vi "TestTactic.vi"(8 "error in (no error)":errorcluster, 9 "Game in":refnum<class "Game.lvclass">, 10 "Robot":refnum<class "Robot.lvclass">, 11 "Tactic in":refnum<class "TestTactic.lvclass">) -> (0 "error out":errorcluster, 2 "Robot out":refnum<class "Robot.lvclass">, 3 "Tactic out":refnum<class "TestTactic.lvclass">)   [LabVIEW 2023, in "TestTactic.lvclass"]
uses:
  TestTactic.lvclass
  C:/Users/ebert/Documents/codes/SSL/repo/SSL_AI/Tactic_class/Tactic.lvclass
  Robot_class/Robot.lvclass
  Game_class/Game.lvclass
  Robot_class/tactics.ctl
  STP_Parameters/TestSkills.ctl
  Tactic_class/Tactic.lvclass/Tactic.ctl
  Game_class/Game.lvclass/Game.ctl
  Team_class/Team.lvclass/Team.ctl
  Robot_class/Robot.lvclass/Robot.ctl
  Game_class/Read BallRef.vi
  Game_class/Read EnemyRef.vi
  Team_class/Read RobotRef.vi
  Tactic_class/Read Skillbook.vi
  Robot_class/Write tactic.vi
  Enemy_class/Enemy.lvclass
  C:/Users/ebert/Documents/codes/SSL/repo/SSL_AI/Team_class/Team.lvclass
  Skillbook_class/Skillbook.lvclass
  Ball_class/Ball.lvclass
  Circulate_class/CirculateSkill.lvclass
  PassSkill_class/PassSkill.lvclass
  OneTouchShotSkill_class/OneTouchShotSkill.lvclass
  AlignSkill/AlignSkill.lvclass
  GoToSkill_v2_class/GoToSkill_v2.lvclass
panel:
  out "x .or. y?":bool
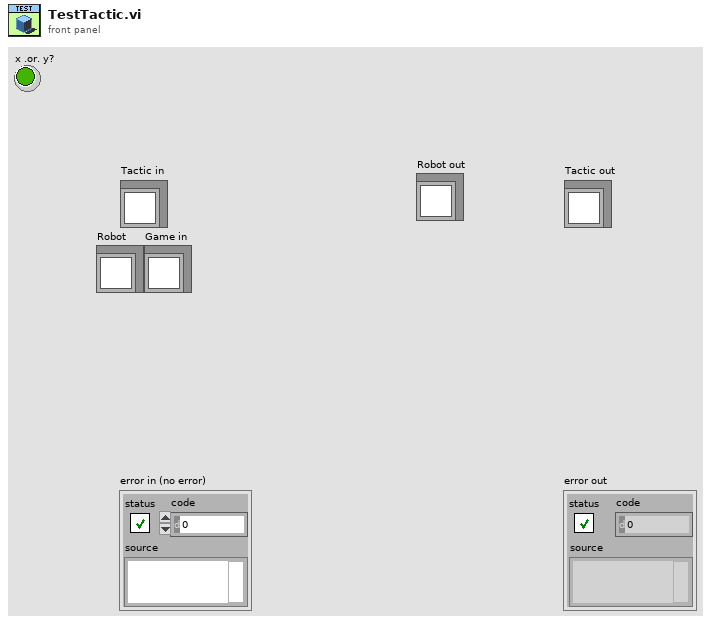
[diagram p1: front panel]
types:
  T1 = typedef "TestSkills.ctl" = enum16{"AlignSkill", "PassSkill", "CirculateBall", "OneTouchShotSkill", "KickToSkill_v2", "ShootSkill", "InterceptBall", "Exit", "GoToSkill_v2"}
  T2 = typedef "tactics.ctl" = enum16{"GoToBallPlacementPosition", "PlaceBall", "GoToBallPlacement", "5Robots", "BallPlacementEnemy", "ReceivePassInFuturePoint", "Roller", "PrepareRollToPassRollerGoTo", "PrepareRollToPassReceiverGoTo", "WaitRoll", "PositionToRoll", "PenaltyAttacker", "PassObserver", "PenaltyDefense", "TableReceiverTactic", "Test", "DefendGoal", "Marker", "FollowAttacker", "DefendArea", "Shoot", "AttackerAimGoal", "AttackerBallOutOfField", "AttackerBlock", "AttackerStop", "Duelist", "Halt", "ZigZag", "GoTo", "Timeout", "KickToBestRobot", "KickToPassReceiver", "PositionToReceivePass", "WaitPass"}
  T3 = typedef "STPParameters.ctl" = cluster{"Skills":T4, "TestSkill":T1, "Events":cluster{"distanceToBallPossession":dbl, "timeForPossessionThreshold":dbl}, "Criteria":cluster{"OpenAngleToGoal":cluster{"minAngle":dbl, "maxAngle":dbl, "minEvaluation":dbl}, "PassDistance":cluster{"maxDistance":dbl, "minDistance":dbl}, "ShotTime":cluster{"shotSpeed":dbl, "keeperSpeed":dbl, "maxShotDistance":dbl, "minEvaluation":dbl}, "OneTouchShot":cluster{"MaxAngle":dbl, "minEvaluation":dbl}, "BallInterception":cluster{"minEnemySpeed":dbl, "maxEnemySpeed":dbl, "chipPassDistance":dbl, "chipPassEval":dbl, "minEvaluation":dbl}}, "minPassSpeed":dbl, "maxPassSpeed":dbl, "AllyTeamIds":T6[]}
  T4 = typedef "Skills.ctl" = cluster{"CirculateBall":T5, "ProtectBall":cluster{"DistanceFromBall":dbl}}
  T5 = typedef "CIrculateSkillParameters.ctl" = cluster{"rotationAngle":dbl, "velocityFactor":dbl, "OrientationFactor":dbl}
  T6 = typedef "AllyTeam.ctl" = enum16{"Keeper", "Defender", "Attacker"}
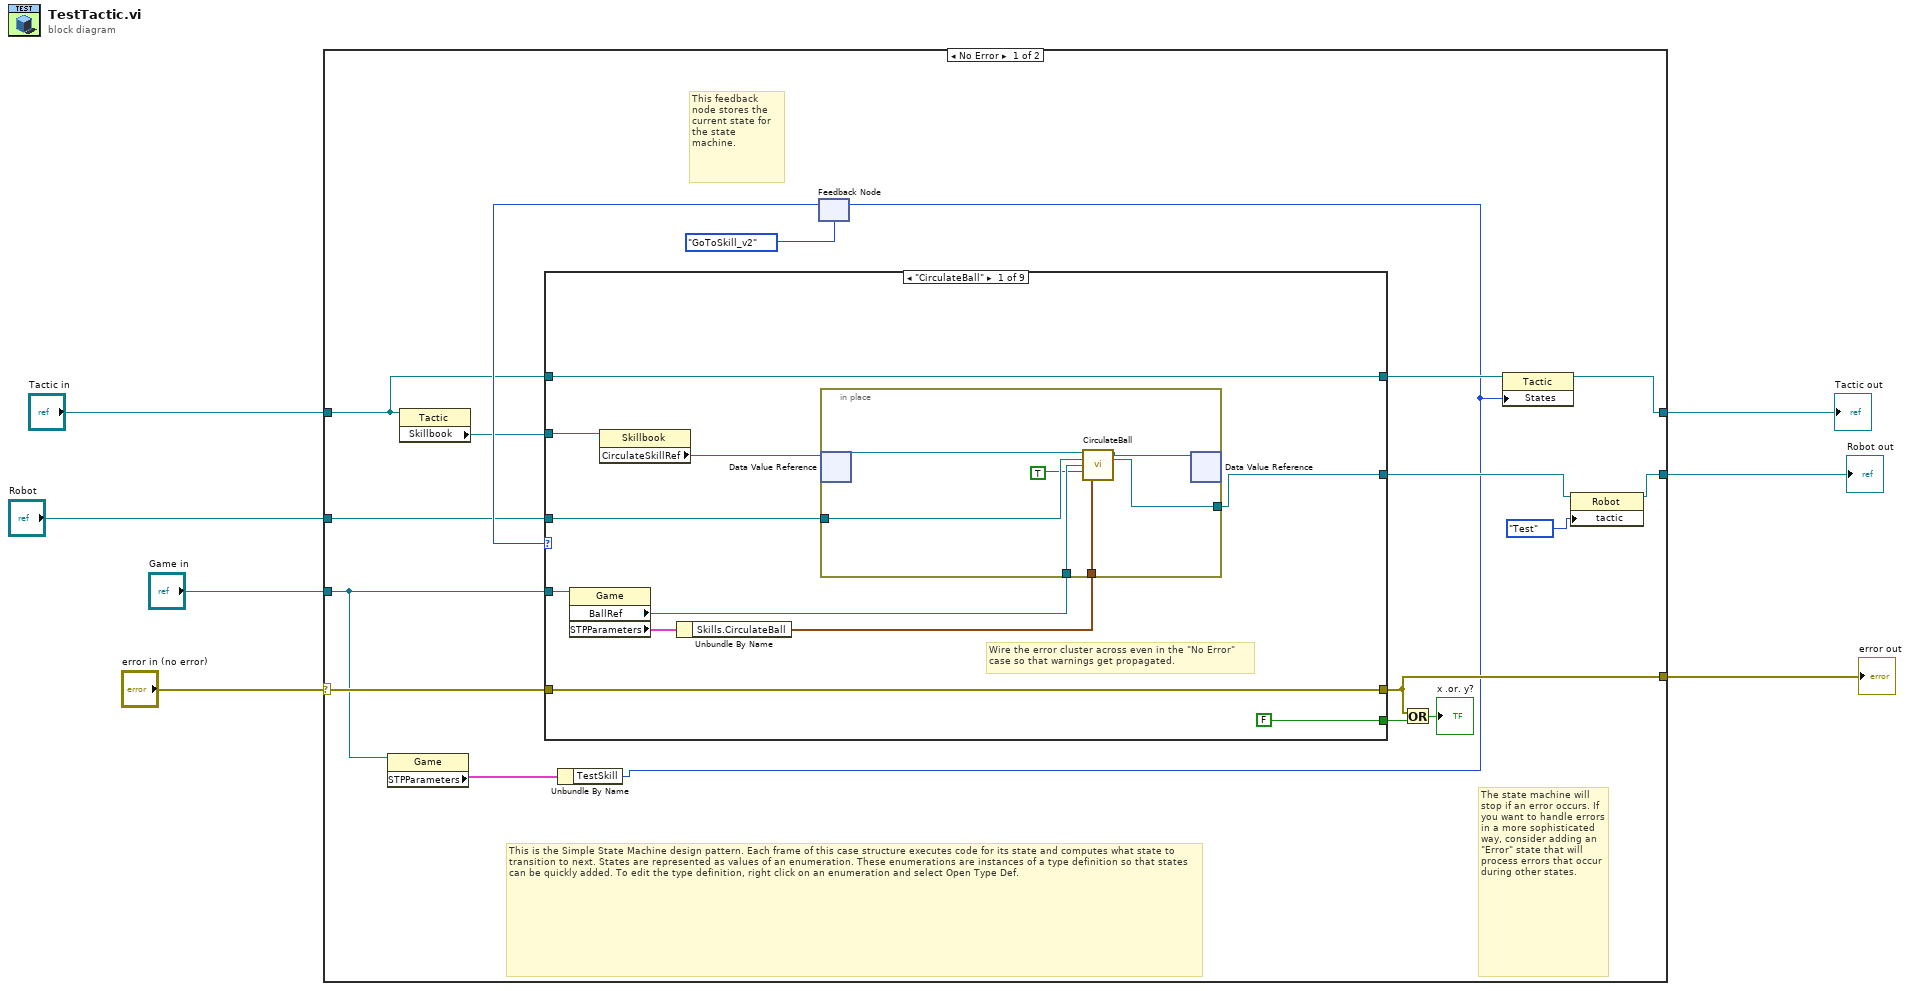
[diagram p0: block diagram]
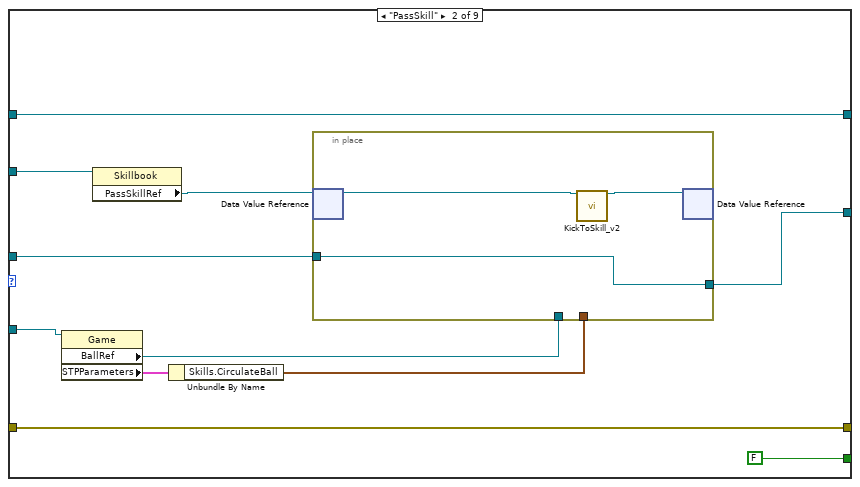
[diagram p2: hidden frame]
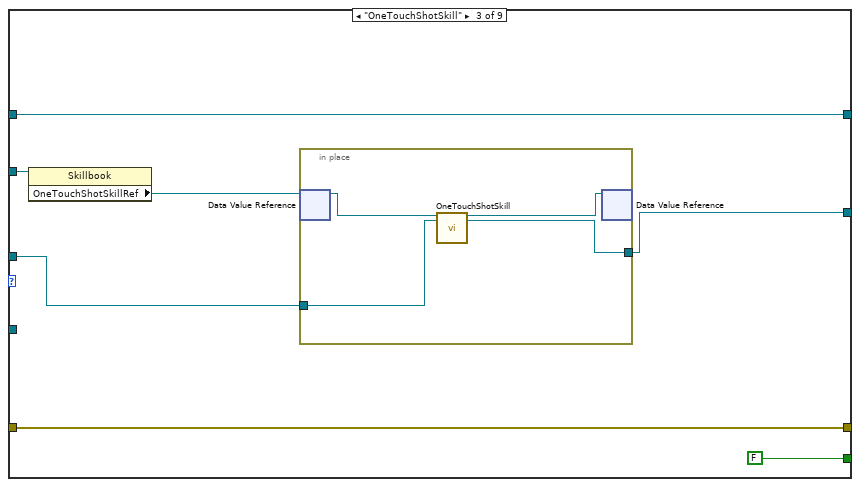
[diagram p3: hidden frame]
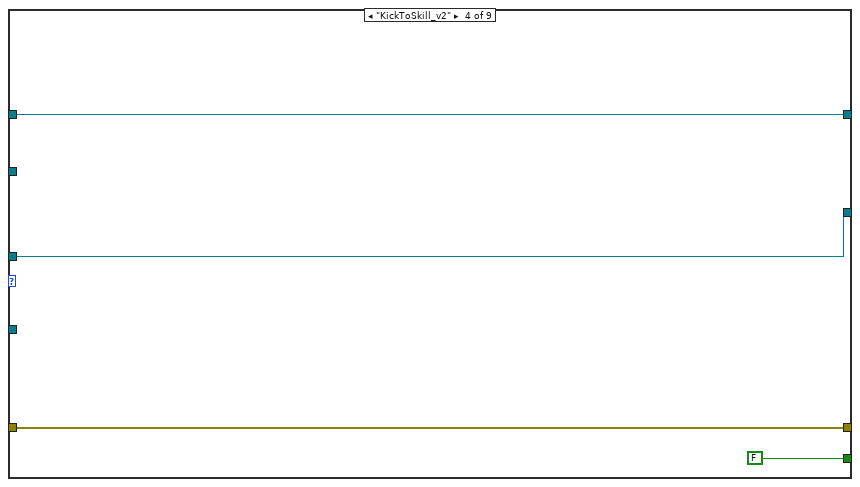
[diagram p4: hidden frame]
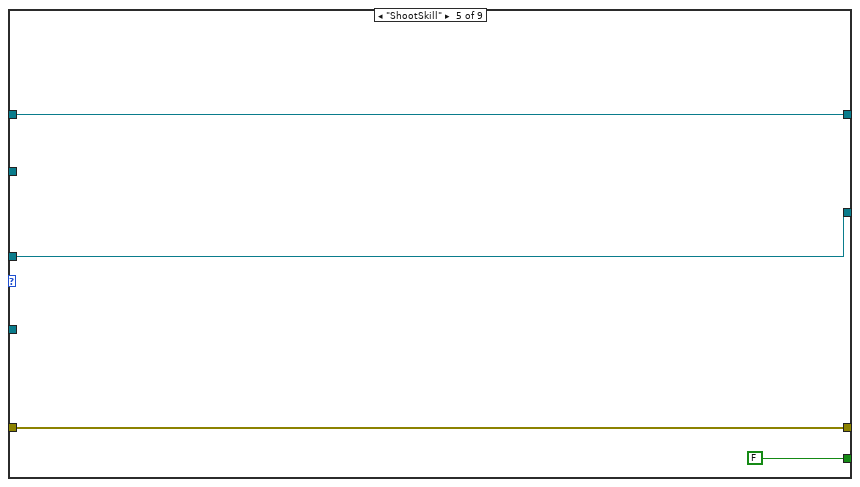
[diagram p5: hidden frame]
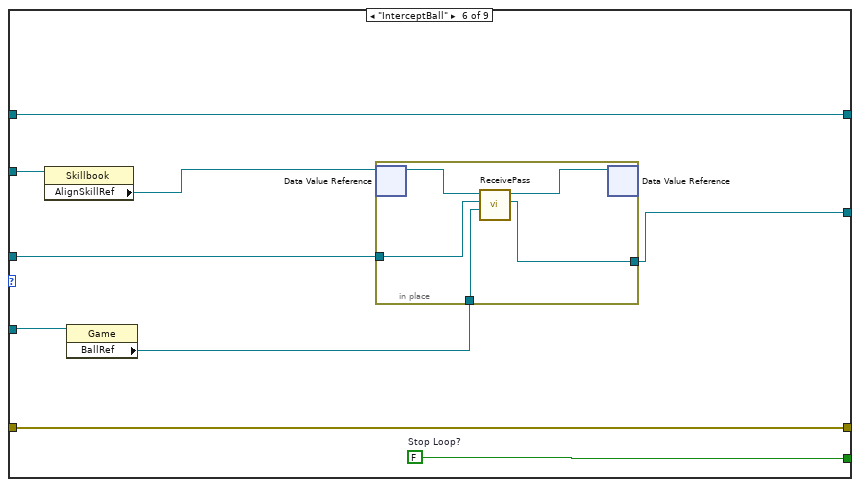
[diagram p6: hidden frame]
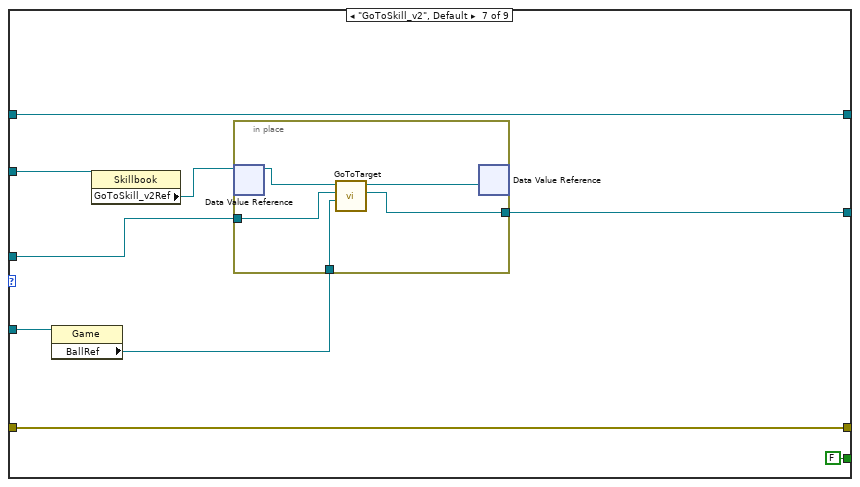
[diagram p7: hidden frame]
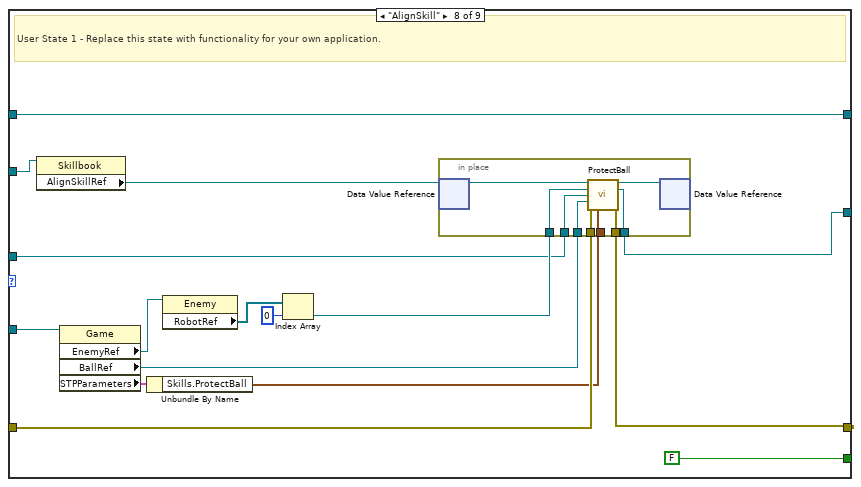
[diagram p8: hidden frame]
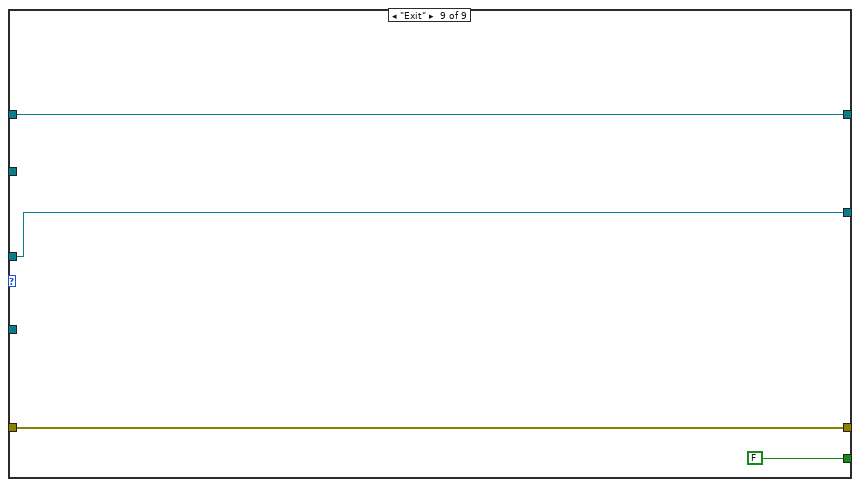
[diagram p9: hidden frame]
diagram:
  n1 = case shown="No Error" "error in (no error)" {
    selector: "error in (no error)" -> [w21 w135]
    tunnel: [w20 w135] -> w6
    tunnel: [w15 w134] -> w5
    tunnel: "Tactic in" -> [w18 w134]
    tunnel: "Robot" -> [w19 w133]
    tunnel: [w12 w133] -> w4
    tunnel: "Game in" -> [w10 _]
    frame No Error {
      # "The state machine will stop if an error occurs. If you want to handle errors in a more sophisticated way, consider adding an \"Error\" state that will process errors that occur during other states."
      # "This feedback node stores the current state for the state machine."
      # "This is the Simple State Machine design pattern. Each frame of this case structure executes code for its state and computes what state to transition to next. States are represented as values of an enumeration. These enumerations are instances of a type definition so that states can be quickly added. To edit the type definition, right click on an enumeration and select Open Type Def."
      # "Wire the error cluster across even in the \"No Error\"\ncase so that warnings get propagated."
      n2 = property class="Game"(reference=w10) -> ("STPParameters"=w9:T3)  [unwired: 1 in, 2 out]
      n3 = property class="Tactic"(reference=w18) -> ("Skillbook"=w17:refnum<class "Skillbook.lvclass">)  [unwired: 1 in, 2 out]
      n4 = Unbundle By Name(w9) -> ("TestSkill"=w8:T1)
      n5 = feedback #1(TestSkills."GoToSkill_v2" ("Enum")) -> (w22:T1)
      n6 = case shown="\"CirculateBall\"" w22 {
        tunnel: [FALSE ("Stop Loop?") FALSE ("Stop Loop?") FALSE ("Stop Loop?") FALSE ("Stop Loop?") FALSE ("Stop Loop?") w83 FALSE ("Stop Loop?") FALSE ("Stop Loop?") FALSE ("Stop Loop?")] -> w24
        tunnel: w21 -> [w35 w53 w63 w71 w75 w84 w98 w107 w132]
        tunnel: [w35 w53 w63 w71 w75 w84 w98 w106 w132] -> w20
        tunnel: w17 -> [w34 w47 w61 _ _ w81 w96 w116 _]
        tunnel: w19 -> [w32 w46 w59 w69 w74 w79 w94 w110 w130]
        tunnel: [w29 w44 w57 w69 w74 w78 w90 w109 w130] -> w13
        tunnel: [w31 w48 w62 w70 w73 w82 w97 w118 w131] -> w16
        tunnel: w18 -> [w31 w48 w62 w70 w73 w82 w97 w118 w131]
        tunnel: w10 -> [w28 w45 _ _ _ w77 w92 w117 _]
        frame "CirculateBall" {
          n7 = property class="Game"(reference=w28) -> ("BallRef"=w27:refnum<class "Ball.lvclass">, "STPParameters"=w26:T3)  [unwired: 1 in, 2 out]
          n8 = property class="Skillbook"(reference=w34) -> ("CirculateSkillRef"=w33:refnum<data-value>)  [unwired: 1 in, 2 out]
          n9 = Unbundle By Name(w26) -> ("Skills.CirculateBall"=w25:T5)
          n10 = in-place {
            in-place-border: w32 -> [w42]
            in-place-border: [w40] -> w29
            in-place-border: w27 -> [w41]
            in-place-border: w25 -> [w36]
            n11 = in-place-dvr #2(w33) -> (w37:refnum<class "CirculateSkill.lvclass">)  [unwired: 1 out]
            n12 = call-dynamic "CirculateBall.vi"("CirculateSkill in"=w37, "Robot"=w42, "BallRef"=w41, "Clockwise?"=TRUE, "Skills.CirculateBall"=w36) -> ("CirculateSkill out"=w39:refnum<class "CirculateSkill.lvclass">, "Robot out"=w40:refnum<class "Robot.lvclass">)  [unwired: 8 in, 1 out]
            n13 = in-place-dvr #2(w39) -> ()  [unwired: 2 out]
          }
        }
        frame "PassSkill" {
          n14 = property class="Game"(reference=w45) -> ("BallRef"=w51:refnum<class "Ball.lvclass">, "STPParameters"=w50:T3)  [unwired: 1 in, 2 out]
          n15 = property class="Skillbook"(reference=w47) -> ("PassSkillRef"=w52:refnum<data-value>)  [unwired: 1 in, 2 out]
          n16 = Unbundle By Name(w50) -> ("Skills.CirculateBall"=w49:T5)
          n17 = in-place {
            in-place-border: w51 -> [_]
            in-place-border: w49 -> [_]
            in-place-border: w46 -> [w54]
            in-place-border: [w54] -> w44
            n18 = in-place-dvr #3(w52) -> (w56:refnum<class "PassSkill.lvclass">)  [unwired: 1 out]
            n19 = call-dynamic "KickToSkill_v2.vi"("object in"=w56) -> ("object out"=w55:refnum<class "PassSkill.lvclass">)  [unwired: 17 in, 1 out]
            n20 = in-place-dvr #3(w55) -> ()  [unwired: 2 out]
          }
        }
        frame "OneTouchShotSkill" {
          n21 = property class="Skillbook"(reference=w61) -> ("OneTouchShotSkillRef"=w60:refnum<data-value>)  [unwired: 1 in, 2 out]
          n22 = in-place {
            in-place-border: w59 -> [w65]
            in-place-border: [w64] -> w57
            n23 = in-place-dvr #4(w60) -> (w67:refnum<class "OneTouchShotSkill.lvclass">)  [unwired: 1 out]
            n24 = call-dynamic "OneTouchShotSkill.vi"("object in"=w67, "Robot in"=w65) -> ("object out"=w66:refnum<class "OneTouchShotSkill.lvclass">, "Robot out"=w64:refnum<class "Robot.lvclass">)  [unwired: 15 in, 1 out]
            n25 = in-place-dvr #4(w66) -> ()  [unwired: 2 out]
          }
        }
        frame "KickToSkill_v2" {
        }
        frame "ShootSkill" {
        }
        frame "InterceptBall" {
          w83 = FALSE  # Stop Loop?
          n26 = property class="Skillbook"(reference=w81) -> ("AlignSkillRef"=w80:refnum<data-value>)  [unwired: 1 in, 2 out]
          n27 = property class="Game"(reference=w77) -> ("BallRef"=w76:refnum<class "Ball.lvclass">)  [unwired: 1 in, 2 out]
          n28 = in-place {
            in-place-border: w79 -> [w89]
            in-place-border: [w86] -> w78
            in-place-border: w76 -> [w85]
            n29 = in-place-dvr #5(w80) -> (w88:refnum<class "AlignSkill.lvclass">)  [unwired: 1 out]
            n30 = call-dynamic "ReceivePass.vi"("Ball"=w85, "Robot in"=w89, "AlignSkill in"=w88) -> ("Robot out"=w86:refnum<class "Robot.lvclass">, "AlignSkill out"=w87:refnum<class "AlignSkill.lvclass">)  [unwired: 6 in, 1 out]
            n31 = in-place-dvr #5(w87) -> ()  [unwired: 2 out]
          }
        }
        frame "GoToSkill_v2", Default {
          n32 = property class="Game"(reference=w92) -> ("BallRef"=w91:refnum<class "Ball.lvclass">)  [unwired: 1 in, 2 out]
          n33 = property class="Skillbook"(reference=w96) -> ("GoToSkill_v2Ref"=w95:refnum<data-value>)  [unwired: 1 in, 2 out]
          n34 = in-place {
            in-place-border: w94 -> [w102]
            in-place-border: w91 -> [w103]
            in-place-border: [w99] -> w90
            n35 = in-place-dvr #6(w95) -> (w101:refnum<class "GoToSkill_v2.lvclass">)  [unwired: 1 out]
            n36 = call-dynamic "GoToTarget.vi"("Ball"=w103, "Robot"=w102, "object in"=w101) -> ("Robot out"=w99:refnum<class "Robot.lvclass">, "object out"=w100:refnum<class "GoToSkill_v2.lvclass">)  [unwired: 6 in, 1 out]
            n37 = in-place-dvr #6(w100) -> ()  [unwired: 2 out]
          }
        }
        frame "AlignSkill" {
          # "User State 1 - Replace this state with functionality for your own application."
          n38 = property class="Skillbook"(reference=w116) -> ("AlignSkillRef"=w108:refnum<data-value>)  [unwired: 1 in, 2 out]
          n39 = property class="Game"(reference=w117) -> ("EnemyRef"=w114:refnum<class "Enemy.lvclass">, "BallRef"=w111:refnum<class "Ball.lvclass">, "STPParameters"=w105:T3)  [unwired: 1 in, 2 out]
          n40 = Unbundle By Name(w105) -> ("Skills.ProtectBall"=w104:cluster{"DistanceFromBall":dbl})
          n41 = property class="Enemy"(reference=w114) -> ("RobotRef"=w115:refnum<class "Robot.lvclass">[])  [unwired: 1 in, 2 out]
          n42 = Index Array(array=w115, index=0) -> (element=w112:refnum<class "Robot.lvclass">)
          n43 = in-place {
            in-place-border: w112 -> [w128]
            in-place-border: w111 -> [w127]
            in-place-border: w110 -> [w126]
            in-place-border: [w125] -> w109
            in-place-border: w107 -> [w122]
            in-place-border: [w121] -> w106
            in-place-border: w104 -> [w120]
            n44 = in-place-dvr #7(w108) -> (w124:refnum<class "AlignSkill.lvclass">)  [unwired: 1 out]
            n45 = call-dynamic "ProtectBall.vi"("AlignSkill in"=w124, "Enemy"=w128, "Robot"=w126, "BallRef"=w127, "error in (no error)"=w122, "Skills.ProtectBall"=w120) -> ("AlignSkill out"=w123:refnum<class "AlignSkill.lvclass">, "Robot out"=w125:refnum<class "Robot.lvclass">, "error out"=w121:errorcluster)  [unwired: 7 in]
            n46 = in-place-dvr #7(w123) -> ()  [unwired: 2 out]
          }
        }
        frame "Exit" {
        }
      }
      n47 = feedback-in #1(w8) -> ()
      n48 = Or(x=w20, y=w24) -> (x .or. y?=→"x .or. y?":bool)
      n49 = property class="Tactic"(reference=w16, "States"=w8) -> (reference out=w15:refnum<class "TestTactic.lvclass">)  [unwired: 1 in, 1 out]
      n50 = property class="Robot"(reference=w13, "tactic"=tactics."Test") -> (reference out=w12:refnum<class "Robot.lvclass">)  [unwired: 1 in, 1 out]
    }
    frame Error {
    }
  }
  "error out" <- w6
  "Tactic out" <- w5
  "Robot out" <- w4
